vi "Time-ConvertStringtoTS.vi"() -> ()   [LabVIEW 2014]
uses:
  ftw-dataflow/ftw/src/core/time/FTW-Time-DisplayFormat-Timestamp.ctl
  <vilib>/addons/database/Connection.llb/DB Tools Open Connec (Path).vi
  <vilib>/addons/database/NI_Database_API.lvlib
panel:
  out "String converted to Time Stamp":timestamp
  in  "String in HH:MM:SS format":string="17:47:00"
  out "Array":string[](array[string])
  out "data":string[][](table)
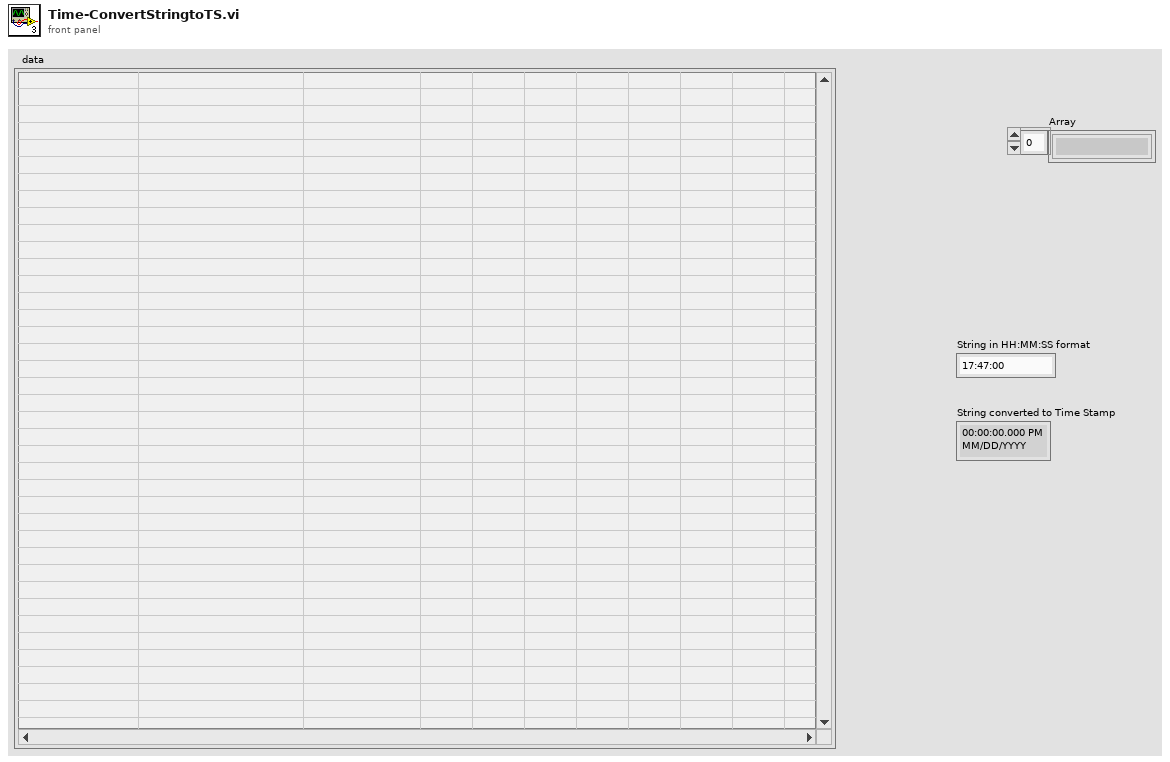
[diagram p1: front panel]
types:
  T1 = typedef "NI_Database_API.lvlib/Conn ObjectReference.ctl" = refnum<k1>
  T2 = typedef "FTW-Time-DisplayFormat-Timestamp.ctl" = enum16{"YYYY-MM-DDT00:00:00.000Z (ISO-8601)", "YYYY-MM-DDT00-00-00Z (Simple ISO-8601)", "YYYY-MM-DD"}
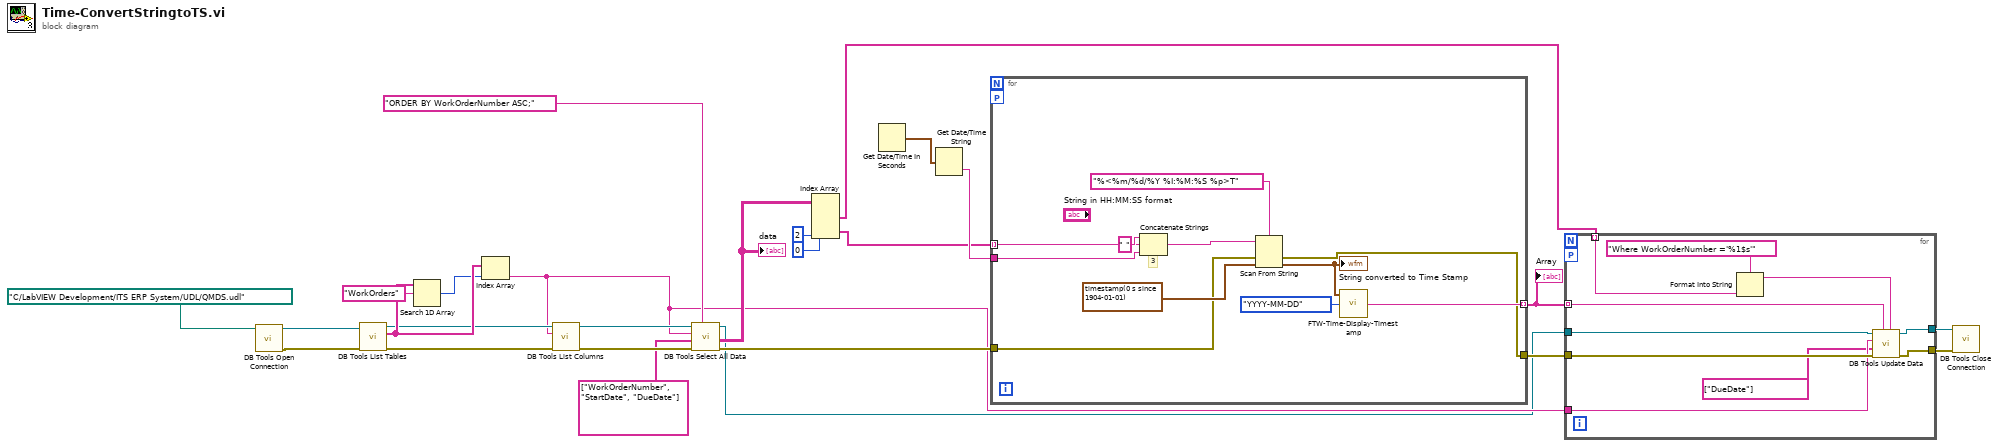
[diagram p0: block diagram]
diagram:
  n1 = call-poly <vilib>:"DB Tools Open Connection.vi"("connection information"=path "C:/LabVIEW Development/ITS ERP System/UDL/QMDS.udl" ("Database (mdb)  File Path")) -> ("error out"=w19:errorcluster, "connection reference"=w18:T1)  [unwired: 7 in]
  n2 = call <vilib>:"DB Tools List Tables.vi"("error in (no error)"=w19, "connection reference"=w18) -> ("error out"=w23:errorcluster, "tables"=w26:string[], "connection reference out"=w24:T1)  [unwired: 3 in]
  n3 = Search 1D Array(1D array=w26, element="WorkOrders") -> (index of element=w25:i32)  [unwired: 1 in]
  n4 = Index Array(array=w26, index=w25) -> (element=w6:string)
  n5 = call <vilib>:"DB Tools List Columns.vi"("error in (no error)"=w23, "table"=w6, "connection reference"=w24) -> ("error out"=w21:errorcluster, "connection reference out"=w22:T1)  [unwired: 1 in, 2 out]
  n6 = call <vilib>:"DB Tools Select All Data.vi"("optional clause"="ORDER BY WorkOrderNumber ASC;" ("SQL Query Statement"), "error in (no error)"=w21, "columns"=string[] ["WorkOrderNumber", "StartDate", "DueDate"], "table"=w6, "connection reference"=w22) -> ("error out"=w11:errorcluster, "data"=w12:string[][], "connection reference out"=w4:T1)  [unwired: 1 in]
  "data" <- w12
  n7 = Index Array(array=w12, index (col) #1=0 ("disabled index (col)"), index (col) #2=2 ("disabled index (col)")) -> (element #1=w7:string[], element #2=w8:string[])  [unwired: 2 in]
  n8 = Get Date/Time In Seconds() -> (seconds since 1Jan1904=w13:timestamp)
  n9 = Get Date/Time String(seconds (now)=w13) -> (time string=w14:string)  [unwired: 2 in, 1 out]
  n10 = for {
    tunnel: w8 -> [w31] mode=indexing
    tunnel: [w33] -> w5 mode=indexing
    tunnel: w14 -> [w29]
    workers-P: _ -> [_]
    tunnel: w11 -> [w28]
    tunnel: [w27] -> w10
    # "3"
    n11 = Concatenate Strings "Concatenate Strings"(w31, " " ("string"), w29) -> (w36:string)
    n12 = Scan From String "Scan From String"(format string="%<%m/%d/%Y %I:%M:%S %p>T" ("input string"), input string=w36, error in=w28, default 1=timestamp(0 s since 1904-01-01) ("default value 1")) -> (error out=w27:errorcluster, output 1=w35:timestamp)  [unwired: 1 in, 2 out]
    "String converted to Time Stamp" <- w35
    n13 = call "FTW-Time-Display-Timestamp.vi"("Format"=FTW-Time-DisplayFormat-Timestamp."YYYY-MM-DD", "Timestamp (unwired for current time)"=w35) -> ("Formatted Timestamp"=w33:string)  [unwired: 2 in]
  }
  "Array" <- w5
  n14 = for {
    tunnel: w10 -> [w47]
    tunnel: w7 -> [w45] mode=indexing
    tunnel: w6 -> [w44]
    tunnel: w5 -> [w42] mode=indexing
    tunnel: w4 -> [w40]
    tunnel: [w39] -> w3
    tunnel: [w38] -> w2
    workers-P: _ -> [_]
    n15 = Format Into String(format string="Where WorkOrderNumber ='%1$s'", w45) -> (resulting string=w41:string)  [unwired: 2 in, 1 out]
    n16 = call <vilib>:"DB Tools Update Data.vi"("condition"=w41, "data"=w42, "error in (no error)"=w47, "columns"=string[] ["DueDate"], "table"=w44, "connection reference"=w40) -> ("error out"=w38:errorcluster, "connection reference out"=w39:T1)  [unwired: 4 in]
  }
  n17 = call <vilib>:"DB Tools Close Connection.vi"("error in (no error)"=w2, "connection reference"=w3) -> ()  [unwired: 5 in, 1 out]
